vi "Save Event Description.vi"(9 "Event Description":string, 11 "Event Ref in":refnum<vi>) -> (0 "error out":errorcluster, 3 "Event Ref out":refnum<vi>)   [LabVIEW 2019, in "Panther Dashboard.lvlib"]
uses:
  Panther Dashboard.lvlib
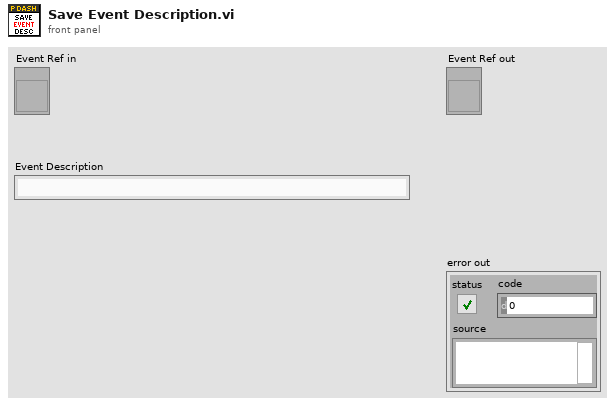
[diagram p1: front panel]
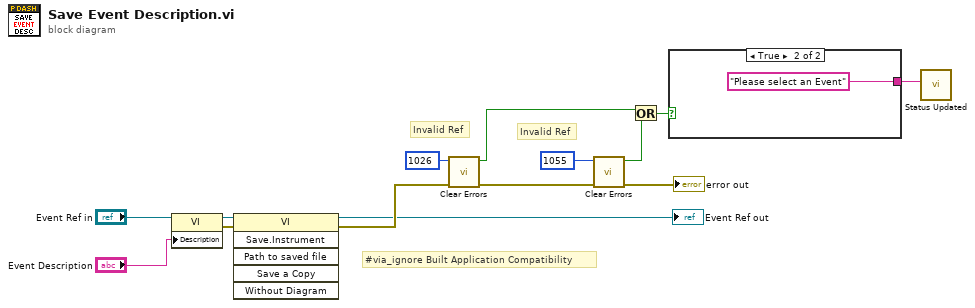
[diagram p0: block diagram]
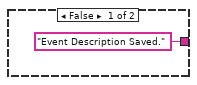
[diagram p2: hidden frame]
diagram:
  # "#via_ignore Built Application Compatibility"
  # "Invalid Ref"
  # "Invalid Ref"
  n1 = property class="VI"(reference="Event Ref in", "Description"="Event Description") -> (reference out=w10:refnum<vi>, error out=w14:errorcluster)  [unwired: 1 in]
  n2 = invoke class="VI" method="Save.Instrument"(reference=w10, error in=w14) -> (reference out=→"Event Ref out":refnum<vi>, error out=w13:errorcluster)  [unwired: 4 in, 4 out]
  n3 = call <vilib>:"Clear Errors.vi"("error in (no error)"=w13, "specific error code to clear (0: all)"=1026) -> ("error out"=w11:errorcluster, "specific error cleared?"=w2:bool)  [unwired: 4 in]
  n4 = call <vilib>:"Clear Errors.vi"("error in (no error)"=w11, "specific error code to clear (0: all)"=1055) -> ("error out"=→"error out":errorcluster, "specific error cleared?"=w9:bool)  [unwired: 4 in]
  n5 = Or(x=w2, y=w9) -> (x .or. y?=w3:bool)
  n6 = case shown="True" w3 {
    tunnel: ["Event Description Saved." ("Status") "Please select an Event" ("Status")] -> w1
    frame False {
    }
    frame True {
    }
  }
  n7 = call "Status Updated.vi"("Status"=w1) -> ()  [unwired: 10 in, 1 out]
